vi "最高權限模式.vi"() -> ()   [LabVIEW 2022 SP3]
panel:
  out "刪除帳密":string[](array[string])
  out "array w/ subset deleted":string[](array[string])
  out "text":string[](array[string])
  out "Tab Control":enum32{"Page 1", "Page 2", "Page 3", "Page 4"}(tab)
  in  "輸入最高權限帳號:":string
  in  "輸入最高權限密碼:":string
  in  "登入":bool
  in  "Stop Button":bool
  in  "選擇帳密儲存位置(txt)":path=path "D:/Project/Semiconductor Equipment/機械手臂/使用者帳密.txt"
  in  "創建使用者帳號":bool
  in  "刪除使用者帳號":bool
  in  "登出":bool
  in  "創建密碼":string
  in  "創建帳號":string
  in  "創建建立":bool
  in  "創建離開":bool
  out "帳號清單":string[](array[string])
  in  "選擇帳號":string(combo)
  in  "刪除離開":bool
  in  "確認刪除":bool
  out "帳號清單":string[](array[string])
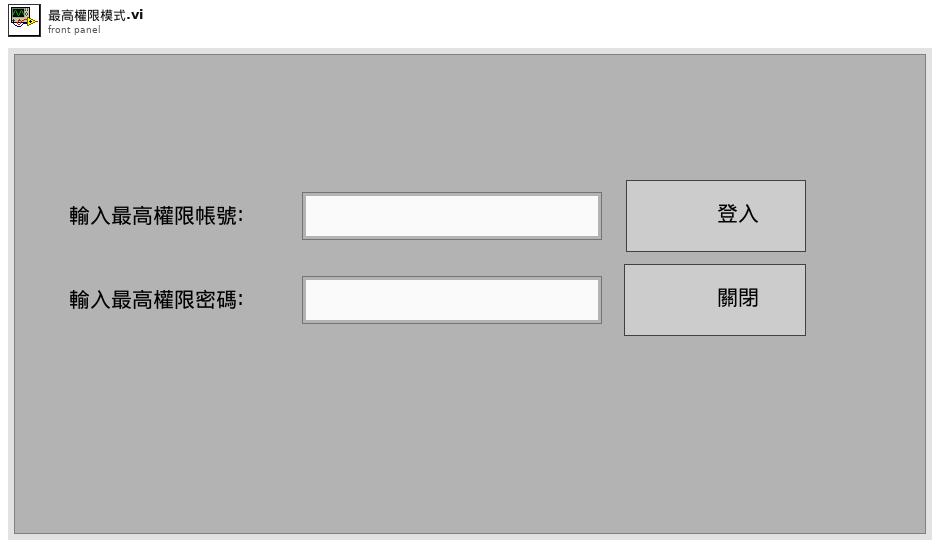
[diagram p1: front panel]
types:
  T1 = typedef "最高權限Control.ctl" = enum16{"刪除寫入", "刪除帳號", "創建帳號", "登出", "登入完成", "初始", "登入", "創建使用者帳密", "刪除使用者帳密", "離開"}
  T2 = enum16{"open", "replace", "create", "open or create", "replace or create", "replace or create with confirmation"}
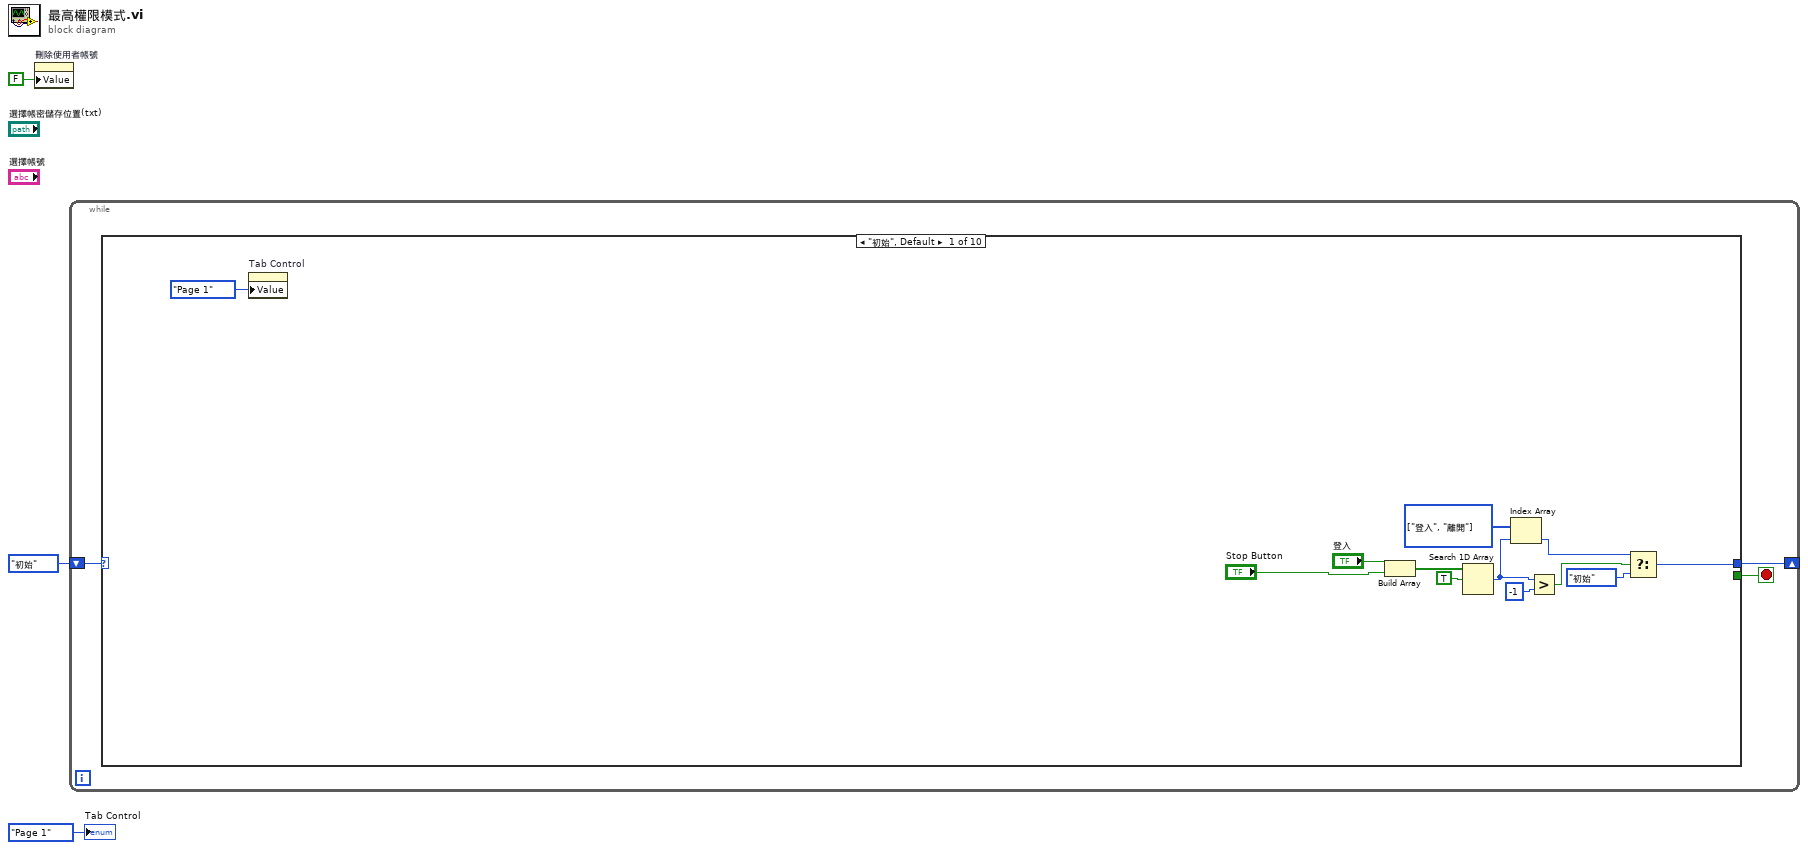
[diagram p0: block diagram]
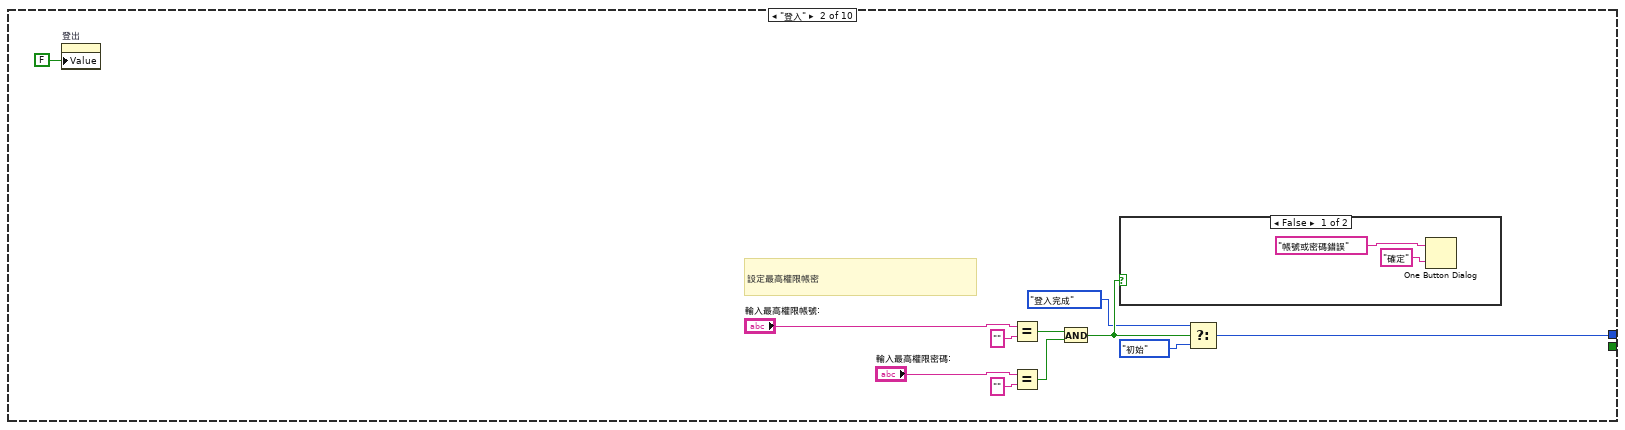
[diagram p2: hidden frame]
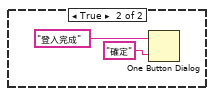
[diagram p3: hidden frame]
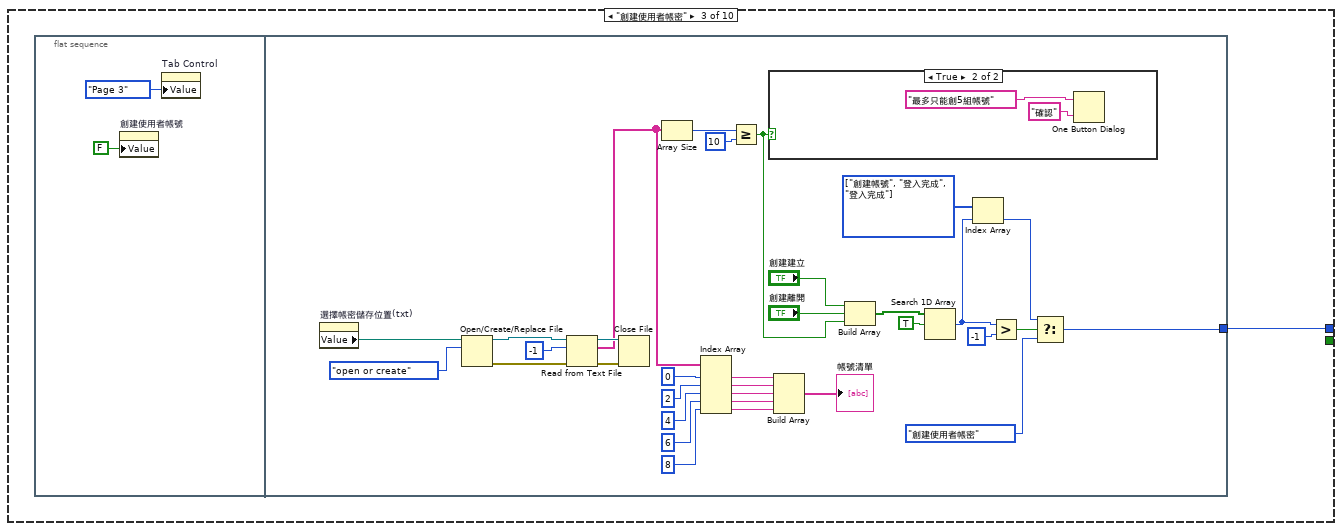
[diagram p4: hidden frame]
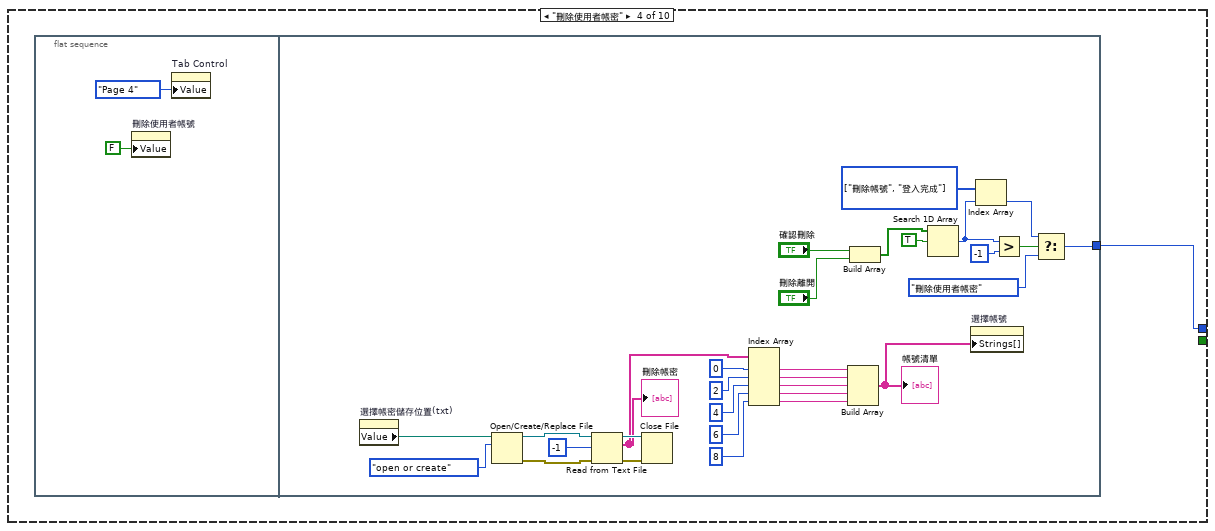
[diagram p6: hidden frame]
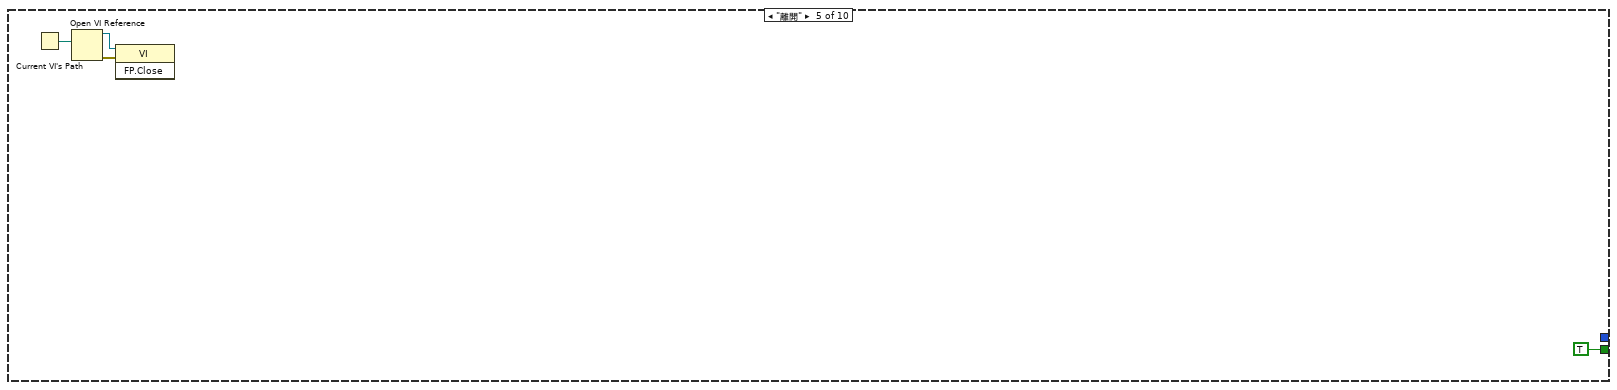
[diagram p7: hidden frame]
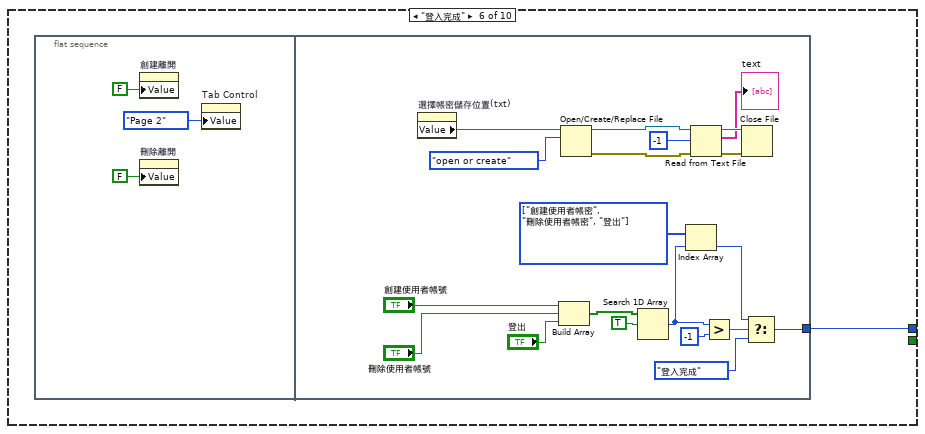
[diagram p8: hidden frame]
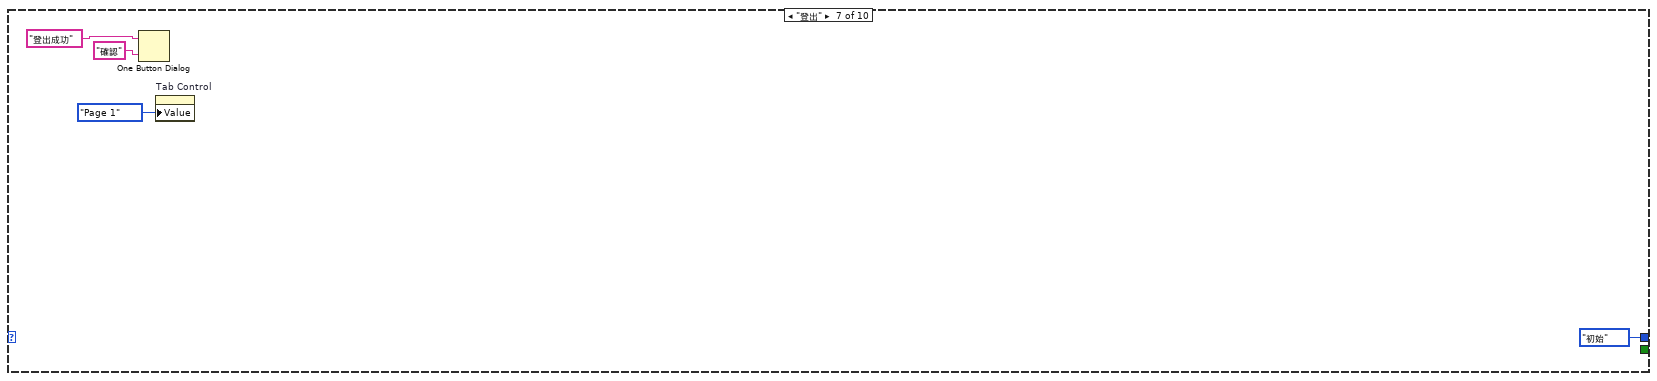
[diagram p9: hidden frame]
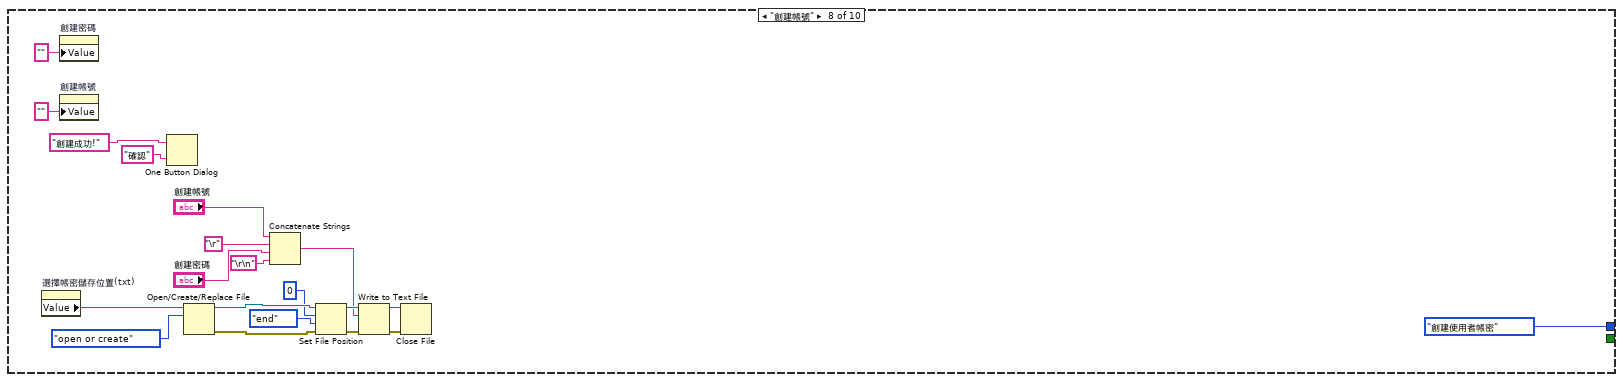
[diagram p10: hidden frame]
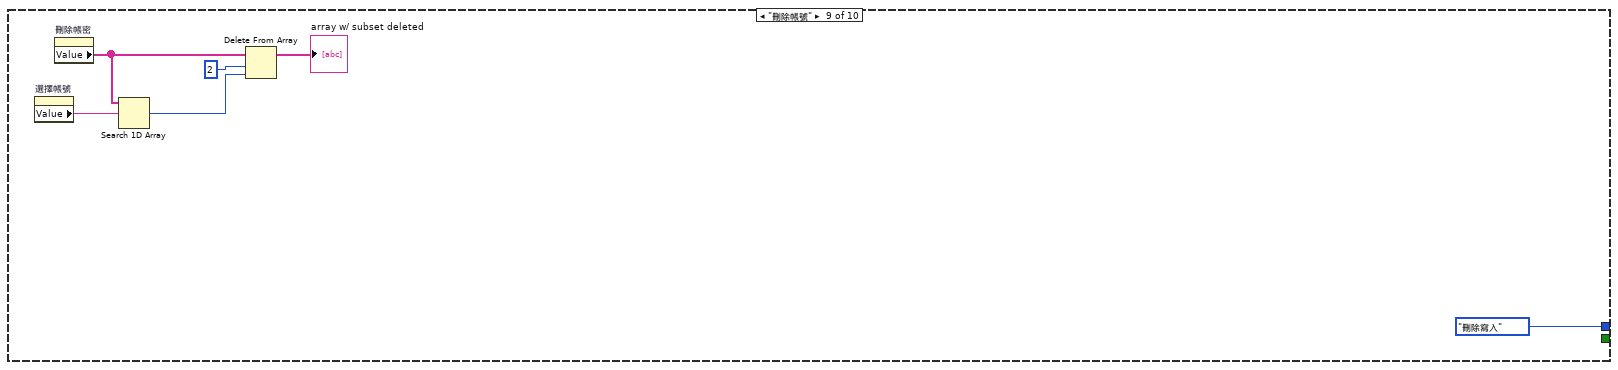
[diagram p11: hidden frame]
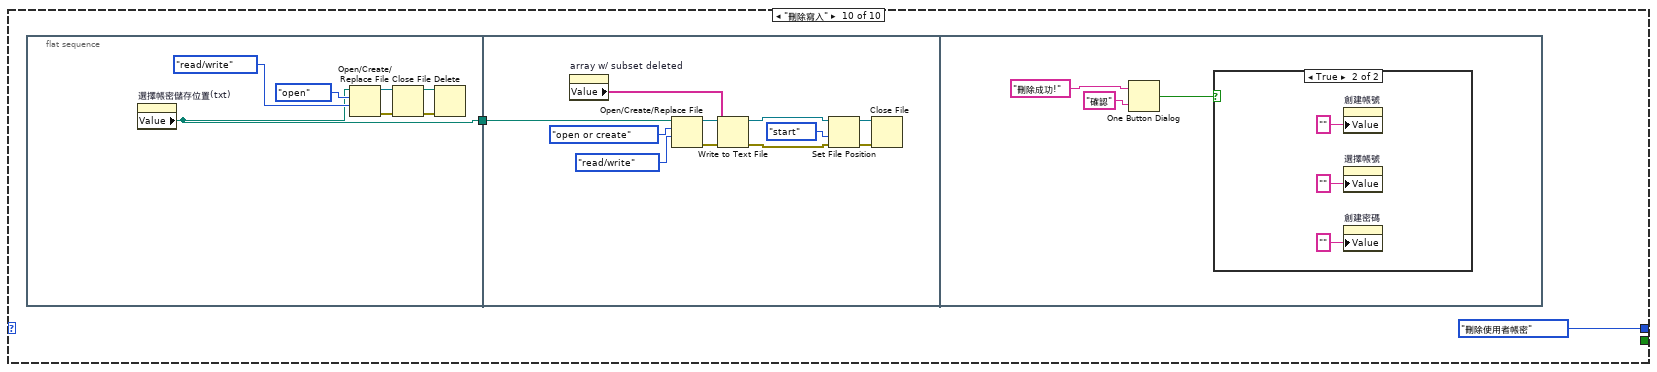
[diagram p12: hidden frame]
diagram:
  n1 = property on="刪除使用者帳號" class="Bool (strict)"("Value"=FALSE ("刪除使用者帳號")) -> ()  [unwired: 2 in, 2 out]
  n2 = while {
    shift-right: [w5] -> _
    shift-left: 最高權限Control."初始" -> [w6]
    stop <- w4 stop-if-true
    n3 = case shown="\"初始\", Default" w6 {
      tunnel: [w9 w20 w34 w72 _ w109 最高權限Control."初始" 最高權限Control."創建使用者帳密" 最高權限Control."刪除寫入" 最高權限Control."刪除使用者帳密"] -> w5
      tunnel: [_ _ _ _ TRUE _ _ _ _ _] -> w4
      frame "初始", Default {
        w14 = T1[] [enum."登入", enum."離開"] items=["刪除寫入", "刪除帳號", "創建帳號", "登出", "登入完成", "初始", "登入", "創建使用者帳密", "刪除使用者帳密", "離開"]
        n4 = property on="Tab Control" class="TabCtl (strict)"("Value"=enum32{"Page 1", "Page 2"}."Page 1" ("Tab Control")) -> ()  [unwired: 2 in, 2 out]
        n5 = Build Array("登入", "Stop Button") -> (w16:bool[])
        n6 = Search 1D Array(1D array=w16, element=TRUE) -> (index of element=w13:i32)  [unwired: 1 in]
        n7 = Index Array(array=w14, index=w13) -> (element=w8:T1)
        n8 = Greater?(x=w13, y=-1) -> (0:w11:bool)
        n9 = Select(t=w8, s=w11, f=最高權限Control."初始") -> (s? t:f=w9:T1)
      }
      frame "登入" {
        # "設定最高權限帳密"
        n10 = property on="登出" class="Bool (strict)"("Value"=FALSE ("登出")) -> ()  [unwired: 2 in, 2 out]
        n11 = Equal?(x="輸入最高權限帳號:", y="") -> (x = y?=w25:bool)
        n12 = Equal?(x="輸入最高權限密碼:", y="") -> (x = y?=w24:bool)
        n13 = And(x=w25, y=w24) -> (x .and. y?=w23:bool)
        n14 = case shown="False" w23 {
          frame False {
            n15 = One Button Dialog(message="帳號或密碼錯誤", button name ("OK")="確定") -> ()  [unwired: 1 out]
          }
          frame True {
            n16 = One Button Dialog(message="登入完成", button name ("OK")="確定") -> ()  [unwired: 1 out]
          }
        }
        n17 = Select(t=最高權限Control."登入完成", s=w23, f=最高權限Control."初始") -> (s? t:f=w20:T1)
      }
      frame "創建使用者帳密" {
        n18 = flat-sequence {
          tunnel: [w59] -> w34
          frame #0 {
            n19 = property on="創建使用者帳號" class="Bool (strict)"("Value"=FALSE ("創建使用者帳號")) -> ()  [unwired: 2 in, 2 out]
            n20 = property on="Tab Control" class="TabCtl (strict)"("Value"=enum32{"Page 1", "Page 2", "Page 3", "Page 4"}."Page 3" ("Tab Control")) -> ()  [unwired: 2 in, 2 out]
          }
          frame #1 {
            w60 = T1[] [enum."創建帳號", enum."登入完成", enum."登入完成"] items=["刪除寫入", "刪除帳號", "創建帳號", "登出", "登入完成", "初始", "登入", "創建使用者帳密", "刪除使用者帳密", "離開"]
            n21 = property on="選擇帳密儲存位置(txt)" class="Path"() -> ("Value"=w37:path)  [unwired: 2 in, 2 out]
            n22 = Open/Create/Replace File(file path (use dialog)=w37, operation (0:open)=T2."open or create") -> (refnum out=w55:refnum<file>, error out=w56:errorcluster)  [unwired: 4 in, 1 out]
            n23 = Read from Text File(file (use dialog)=w55, count=-1, error in=w56) -> (refnum out=w58:refnum<file>, text=w49:string[], error out=w57:errorcluster)  [unwired: 1 in, 1 out]
            n24 = Close File(refnum=w58, error in=w57) -> ()  [unwired: 2 out]
            n25 = Array Size(array=w49) -> (size(s)=w52:i32)
            n26 = Index Array(array=w49, index #1=0 ("index"), index #2=2 ("index"), index #3=4 ("index"), index #4=6 ("index"), index #5=8 ("index")) -> (element #1=w40:string, element #2=w41:string, element #3=w42:string, element #4=w38:string, element #5=w43:string)
            n27 = Greater Or Equal?(x=w52, y=10) -> (x >= y?=w50:bool)
            n28 = case shown="True" w50 {
              frame False {
              }
              frame True {
                n29 = One Button Dialog(message="最多只能創5組帳號", button name ("OK")="確認") -> ()  [unwired: 1 out]
              }
            }
            n30 = Build Array(w40, w41, w42, w38, w43) -> (→"帳號清單":string[])
            n31 = Build Array("創建建立", "創建離開", w50) -> (w69:bool[])
            n32 = Search 1D Array(1D array=w69, element=TRUE) -> (index of element=w68:i32)  [unwired: 1 in]
            n33 = Index Array(array=w60, index=w68) -> (element=w66:T1)
            n34 = Greater?(x=w68, y=-1) -> (0:w67:bool)
            n35 = Select(t=w66, s=w67, f=最高權限Control."創建使用者帳密") -> (s? t:f=w59:T1)
          }
        }
      }
      frame "刪除使用者帳密" {
        n36 = flat-sequence {
          tunnel: [w94] -> w72
          frame #0 {
            n37 = property on="刪除使用者帳號" class="Bool (strict)"("Value"=FALSE ("刪除使用者帳號")) -> ()  [unwired: 2 in, 2 out]
            n38 = property on="Tab Control" class="TabCtl (strict)"("Value"=enum32{"Page 1", "Page 2", "Page 3", "Page 4"}."Page 4" ("Tab Control")) -> ()  [unwired: 2 in, 2 out]
          }
          frame #1 {
            w95 = T1[] [enum."刪除帳號", enum."登入完成"] items=["刪除寫入", "刪除帳號", "創建帳號", "登出", "登入完成", "初始", "登入", "創建使用者帳密", "刪除使用者帳密", "離開"]
            n39 = property on="選擇帳密儲存位置(txt)" class="Path"() -> ("Value"=w75:path)  [unwired: 2 in, 2 out]
            n40 = Open/Create/Replace File(file path (use dialog)=w75, operation (0:open)=T2."open or create") -> (refnum out=w90:refnum<file>, error out=w91:errorcluster)  [unwired: 4 in, 1 out]
            n41 = Read from Text File(file (use dialog)=w90, count=-1, error in=w91) -> (refnum out=w93:refnum<file>, text=w77:string[], error out=w92:errorcluster)  [unwired: 1 in, 1 out]
            "刪除帳密" <- w77
            n42 = Close File(refnum=w93, error in=w92) -> ()  [unwired: 2 out]
            n43 = Index Array(array=w77, index #1=0 ("index"), index #2=2 ("index"), index #3=4 ("index"), index #4=6 ("index"), index #5=8 ("index")) -> (element #1=w86:string, element #2=w87:string, element #3=w88:string, element #4=w85:string, element #5=w89:string)
            n44 = Build Array(w86, w87, w88, w85, w89) -> (w76:string[])
            "帳號清單" <- w76
            n45 = Build Array("確認刪除", "刪除離開") -> (w101:bool[])
            n46 = Search 1D Array(1D array=w101, element=TRUE) -> (index of element=w102:i32)  [unwired: 1 in]
            n47 = property on="選擇帳號" class="CmbBox"("Strings[]"=w76) -> ()  [unwired: 2 in, 2 out]
            n48 = Index Array(array=w95, index=w102) -> (element=w104:T1)
            n49 = Greater?(x=w102, y=-1) -> (0:w103:bool)
            n50 = Select(t=w104, s=w103, f=最高權限Control."刪除使用者帳密") -> (s? t:f=w94:T1)
          }
        }
      }
      frame "離開" {
        n51 = Current VI's Path() -> (path=w105:path)
        n52 = Open VI Reference(vi path=w105) -> (vi reference=w107:refnum<vi>, error out=w106:errorcluster)  [unwired: 5 in]
        n53 = invoke class="VI" method="FP.Close"(reference=w107, error in=w106) -> ()  [unwired: 1 in, 3 out]
      }
      frame "登入完成" {
        n54 = flat-sequence {
          tunnel: [w121] -> w109
          frame #0 {
            n55 = property on="創建離開" class="Bool (strict)"("Value"=FALSE ("創建離開")) -> ()  [unwired: 2 in, 2 out]
            n56 = property on="刪除離開" class="Bool (strict)"("Value"=FALSE ("刪除離開")) -> ()  [unwired: 2 in, 2 out]
            n57 = property on="Tab Control" class="TabCtl (strict)"("Value"=enum32{"Page 1", "Page 2"}."Page 2" ("Tab Control")) -> ()  [unwired: 2 in, 2 out]
          }
          frame #1 {
            w122 = T1[] [enum."創建使用者帳密", enum."刪除使用者帳密", enum."登出"] items=["刪除寫入", "刪除帳號", "創建帳號", "登出", "登入完成", "初始", "登入", "創建使用者帳密", "刪除使用者帳密", "離開"]
            n58 = property on="選擇帳密儲存位置(txt)" class="Path"() -> ("Value"=w113:path)  [unwired: 2 in, 2 out]
            n59 = Build Array("創建使用者帳號", "刪除使用者帳號", "登出") -> (w129:bool[])
            n60 = Open/Create/Replace File(file path (use dialog)=w113, operation (0:open)=T2."open or create") -> (refnum out=w117:refnum<file>, error out=w118:errorcluster)  [unwired: 4 in, 1 out]
            n61 = Search 1D Array(1D array=w129, element=TRUE) -> (index of element=w130:i32)  [unwired: 1 in]
            n62 = Index Array(array=w122, index=w130) -> (element=w131:T1)
            n63 = Read from Text File(file (use dialog)=w117, count=-1, error in=w118) -> (refnum out=w120:refnum<file>, text=→"text":string[], error out=w119:errorcluster)  [unwired: 1 in, 1 out]
            n64 = Greater?(x=w130, y=-1) -> (0:w132:bool)
            n65 = Close File(refnum=w120, error in=w119) -> ()  [unwired: 2 out]
            n66 = Select(t=w131, s=w132, f=最高權限Control."登入完成") -> (s? t:f=w121:T1)
          }
        }
      }
      frame "登出" {
        n67 = One Button Dialog(message="登出成功", button name ("OK")="確認") -> ()  [unwired: 1 out]
        n68 = property on="Tab Control" class="TabCtl (strict)"("Value"=enum32{"Page 1", "Page 2"}."Page 1" ("Tab Control")) -> ()  [unwired: 2 in, 2 out]
      }
      frame "創建帳號" {
        n69 = property on="選擇帳密儲存位置(txt)" class="Path"() -> ("Value"=w137:path)  [unwired: 2 in, 2 out]
        n70 = property on="創建密碼" class="Str"("Value"="" ("創建密碼")) -> ()  [unwired: 2 in, 2 out]
        n71 = property on="創建帳號" class="Str"("Value"="" ("創建帳號")) -> ()  [unwired: 2 in, 2 out]
        n72 = One Button Dialog(message="創建成功!", button name ("OK")="確認") -> ()  [unwired: 1 out]
        n73 = Open/Create/Replace File(file path (use dialog)=w137, operation (0:open)=T2."open or create") -> (refnum out=w149:refnum<file>, error out=w147:errorcluster)  [unwired: 4 in, 1 out]
        n74 = Concatenate Strings("創建帳號", "\r", "創建密碼", "\r\n") -> (w140:string)
        n75 = Set File Position(offset (in bytes) (0)=i64 0, refnum=w149, from (0:start)=enum16{"start", "end", "current"}."end", error in=w147) -> (refnum out=w148:refnum<file>, error out=w146:errorcluster)
        n76 = Write to Text File(file (use dialog)=w148, text=w140, error in=w146) -> (refnum out=w152:refnum<file>, error out=w153:errorcluster)  [unwired: 1 in, 1 out]
        n77 = Close File(refnum=w152, error in=w153) -> ()  [unwired: 2 out]
      }
      frame "刪除帳號" {
        n78 = property on="選擇帳號" class="CmbBox"() -> ("Value"=w158:string)  [unwired: 2 in, 2 out]
        n79 = property on="刪除帳密" class="Arr (strict)"() -> ("Value"=w157:string[])  [unwired: 2 in, 2 out]
        n80 = Search 1D Array(1D array=w157, element=w158) -> (index of element=w161:i32)  [unwired: 1 in]
        n81 = Delete From Array(array=w157, length=2, index=w161) -> (array with subset deleted=→"array w/ subset deleted":string[])  [unwired: 1 out]
      }
      frame "刪除寫入" {
        n82 = flat-sequence {
          tunnel: [w165] -> w163
          tunnel: w163 -> [w172]
          frame #0 {
            n83 = property on="選擇帳密儲存位置(txt)" class="Path"() -> ("Value"=w165:path)  [unwired: 2 in, 2 out]
            n84 = Open/Create/Replace File(file path (use dialog)=w165, operation (0:open)=T2."open", access (0:read/write)=enum16{"read/write", "read-only", "write-only"}."read/write") -> (refnum out=w169:refnum<file>, error out=w168:errorcluster)  [unwired: 3 in, 1 out]
            n85 = Close File(refnum=w169, error in=w168) -> (path=w167:path, error out=w166:errorcluster)
            n86 = Delete(path (use dialog)=w167, error in=w166) -> ()  [unwired: 3 in, 3 out]
          }
          frame #1 {
            n87 = property on="array w/ subset deleted" class="Arr (strict)"() -> ("Value"=w173:string[])  [unwired: 2 in, 2 out]
            n88 = Open/Create/Replace File(file path (use dialog)=w172, operation (0:open)=T2."open or create", access (0:read/write)=enum16{"read/write", "read-only", "write-only"}."read/write") -> (refnum out=w174:refnum<file>, error out=w181:errorcluster)  [unwired: 3 in, 1 out]
            n89 = Write to Text File(file (use dialog)=w174, text=w173, error in=w181) -> (refnum out=w179:refnum<file>, error out=w178:errorcluster)  [unwired: 1 in, 1 out]
            n90 = Set File Position(refnum=w179, from (0:start)=enum16{"start", "end", "current"}."start", error in=w178) -> (refnum out=w176:refnum<file>, error out=w177:errorcluster)  [unwired: 1 in]
            n91 = Close File(refnum=w176, error in=w177) -> ()  [unwired: 2 out]
          }
          frame #2 {
            n92 = One Button Dialog(message="刪除成功!", button name ("OK")="確認") -> (true=w185:bool)
            n93 = case shown="True" w185 {
              frame False {
              }
              frame True {
                n94 = property on="創建帳號" class="Str"("Value"="" ("創建帳號")) -> ()  [unwired: 2 in, 2 out]
                n95 = property on="選擇帳號" class="CmbBox"("Value"="") -> ()  [unwired: 2 in, 2 out]
                n96 = property on="創建密碼" class="Str"("Value"="" ("創建密碼")) -> ()  [unwired: 2 in, 2 out]
              }
            }
          }
        }
      }
    }
  }
  "Tab Control" <- enum32{"Page 1", "Page 2"}."Page 1" ("Tab Control")
